vi "GetNumberOfDigitsOnLHS.vi"(8 "error in (no error)":errorcluster, 11 "UPC in":refnum<class "UPC.lvclass">) -> (0 "error out":errorcluster, 2 "NumberOfDigitsOnLHS":u8=5, 3 "UPC out":refnum<class "UPC.lvclass">)   [LabVIEW 2013, in "BarCodes.lvlib" / "UPC.lvclass"]
uses:
  UPC.lvclass
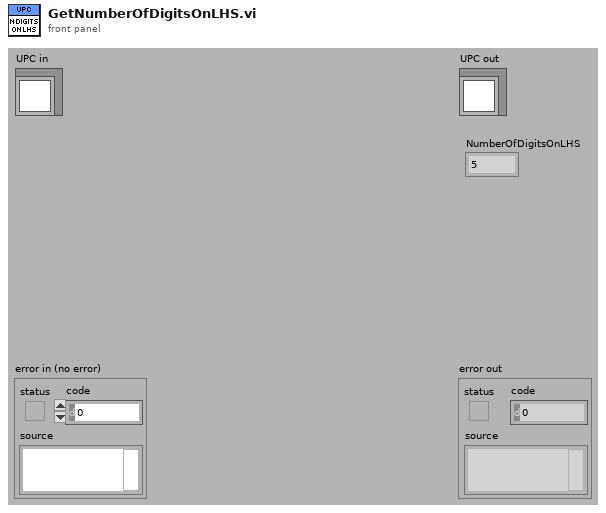
[diagram p1: front panel]
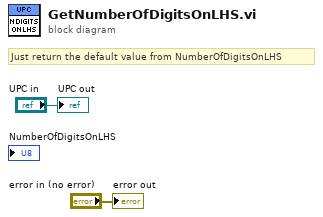
[diagram p0: block diagram]
diagram:
  # "Just return the default value from NumberOfDigitsOnLHS"
  "error out" <- "error in (no error)"
  "UPC out" <- "UPC in"
